vi "ADO Connection Execute.vi"(8 "error in (no error)":errorcluster, 10 "CommandText":string, 11 "ADODB._Connection In":refnum<k7>) -> (0 "error out":errorcluster, 2 "RecordSet":refnum<k7>, 3 "ADODB._Connection Out":refnum<k7>)   [LabVIEW 2013]
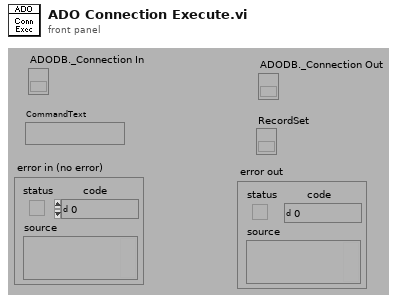
[diagram p1: front panel]
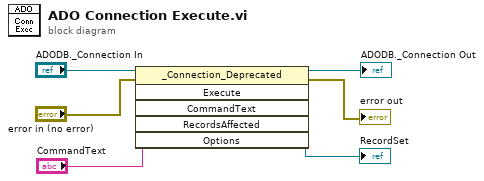
[diagram p0: block diagram]
diagram:
  n1 = invoke class="_Connection_Deprecated" method="Execute"(reference="ADODB._Connection In", error in="error in (no error)", "CommandText"="CommandText") -> (reference out=→"ADODB._Connection Out":refnum<k7>, error out=→"error out":errorcluster, "Execute"=→"RecordSet":refnum<k7>)  [unwired: 3 in, 3 out]
